vi "UNBILITZ-ShutterDriver-Close.vi"(0 "VISA resource name":refnum<visa-resource-name>, 11 "error in (no error)":errorcluster) -> (15 "error out":errorcluster)   [LabVIEW 8.6]
doc: "Closes the serial connection to the Uniblitz shutter driver device."
panel:
  # "Inputs"
  # "Outputs"
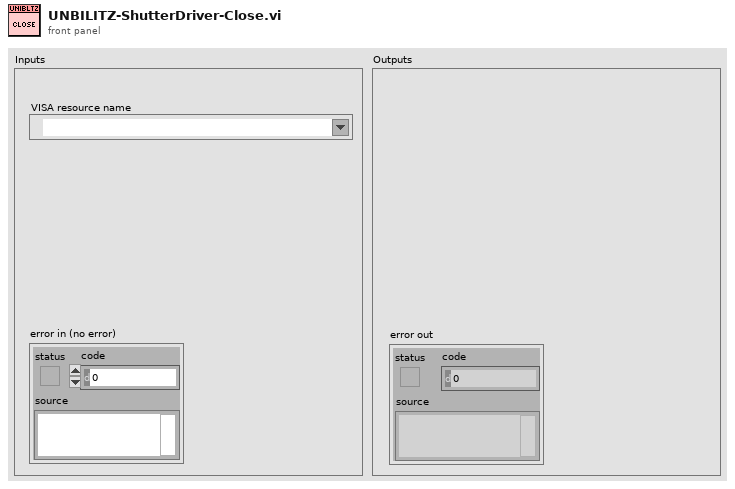
[diagram p1: front panel]
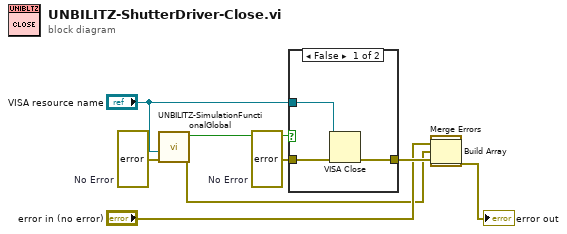
[diagram p0: block diagram]
diagram:
  w2 = errorcluster ?  # No Error
  w5 = errorcluster ?  # No Error
  n1 = call "UNBILITZ-SimulationFunctionalGlobal.vi"("error in (no error)"=w5, "VISA Resource Name"="VISA resource name") -> ("error out"=w3:errorcluster, "Simulation Mode"=w7:bool)  [unwired: 8 in]
  n2 = case shown="False" w7 {
    tunnel: w2 -> [w10 w13]
    tunnel: [w12 w13] -> w9
    tunnel: "VISA resource name" -> [w11 _]
    frame #0 {
      n3 = VISA Close(VISA resource name=w11, error in (no error)=w10) -> (error out=w12:errorcluster)
    }
    frame #1 {
    }
  }
  n4 = Build Array("error in (no error)", w3, w9) -> (w1:errorcluster[])
  n5 = call <vilib>:"Merge Errors.vi"("error array in"=w1) -> ("error out"=→"error out":errorcluster)  [unwired: 6 in]
